vi "Untitled 1.vi"() -> ()   [LabVIEW 2022 SP3]
panel:
  in  "stop":bool
  in  "Boolean 2":bool
  out "Boolean":bool
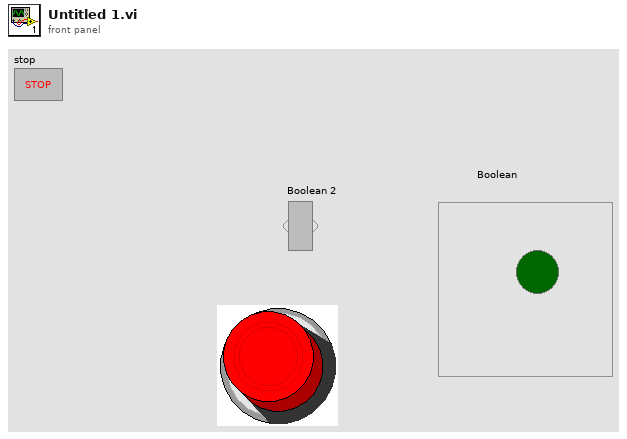
[diagram p1: front panel]
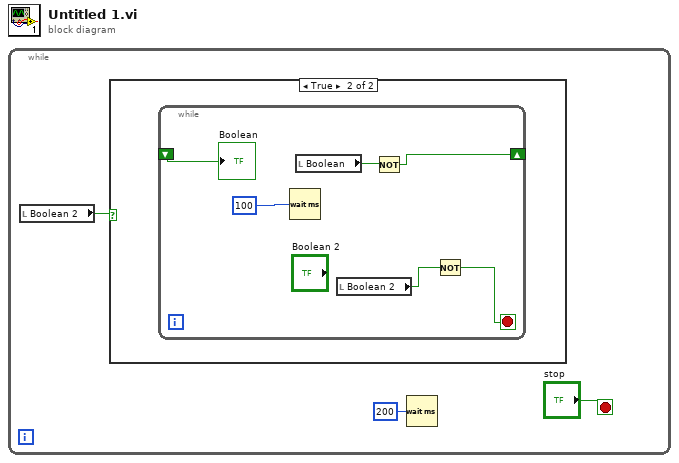
[diagram p0: block diagram]
diagram:
  n1 = while {
    stop <- "stop" stop-if-true
    n2 = local read "Boolean 2"() -> (w2:bool)
    n3 = case shown="True" w2 {
      frame False {
      }
      frame True {
        n4 = while {
          shift-right: [w8] -> _
          shift-left: _ -> [w7]
          stop <- w4 stop-if-true
          n5 = Wait (ms)(milliseconds to wait=u32 100) -> ()  [unwired: 1 out]
          n6 = local read "Boolean"() -> (w9:bool)
          n7 = local read "Boolean 2"() -> (w5:bool)
          n8 = Not(x=w9) -> (.not. x?=w8:bool)
          n9 = Not(x=w5) -> (.not. x?=w4:bool)
          "Boolean" <- w7
        }
      }
    }
    n10 = Wait (ms)(milliseconds to wait=u32 200) -> ()  [unwired: 1 out]
  }
